vi "UpConvert.vi"(5 "clock x2":refnum<k21>="Daughterboard 0\\Data Clock x2", 7 "reset":bool, 8 "input valid":bool, 10 "output sample rate":fxp<+,48,1>, 11 "data in":T1[](array[typedef])=[{"I"=0.0, "Q"=0.0, "overflow"=FALSE}, {"I"=0.0, "Q"=0.0, "overflow"=FALSE}, {"I"=0.0, "Q"=0.0, "overflow"=FALSE}, {"I"=0.0, "Q"=0.0, "overflow"=FALSE}]) -> (0 "output valid":bool, 3 "data out":T1[](array[typedef]))   [LabVIEW 2025]
uses:
  <instrlib>/_niInstr/DSP/v1/FPGA/niInstr DSP v1 FPGA.lvlib
  <instrlib>/_niInstr/DSP/v1/Shared/Public/IQ Data.ctl
  <instrlib>/_niInstr/DSP/v1/Shared/niInstr DSP v1 Shared.lvlib
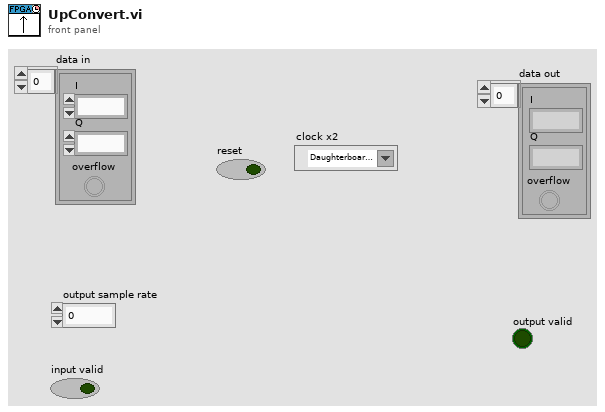
[diagram p1: front panel]
types:
  T1 = typedef "niInstr DSP v1 Shared.lvlib/IQ Data.ctl" = cluster{"I":fxp<+/-,18,1>, "Q":fxp<+/-,18,1>, "overflow":bool}
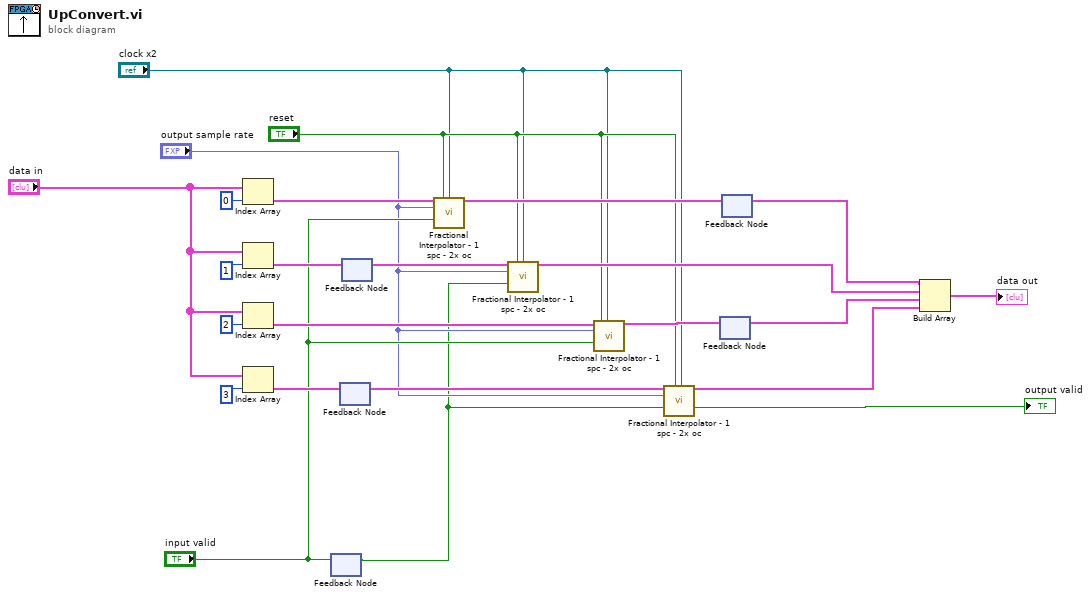
[diagram p0: block diagram]
diagram:
  n1 = Index Array(array="data in", index=0) -> (element=w14:T1)
  n2 = Index Array(array="data in", index=1) -> (element=w19:T1)
  n3 = Index Array(array="data in", index=2) -> (element=w10:T1)
  n4 = Index Array(array="data in", index=3) -> (element=w18:T1)
  n5 = feedback #1() -> (w5:bool)  [unwired: 1 in]
  n6 = feedback-in #1("input valid") -> ()
  n7 = feedback #2() -> (w7:T1)  [unwired: 1 in]
  n8 = feedback-in #2(w18) -> ()
  n9 = feedback #3() -> (w12:T1)  [unwired: 1 in]
  n10 = feedback-in #3(w19) -> ()
  n11 = call <instrlib>:"Fractional Interpolator - 1 spc - 2x oc.vi"("data in"=w14, "reset"="reset", "clock x 2"="clock x2", "input sample rate"="output sample rate", "input valid"="input valid") -> ("data out"=w13:T1)  [unwired: 7 in, 3 out]
  n12 = call <instrlib>:"Fractional Interpolator - 1 spc - 2x oc.vi"("data in"=w12, "reset"="reset", "clock x 2"="clock x2", "input sample rate"="output sample rate", "input valid"=w5) -> ("data out"=w11:T1)  [unwired: 7 in, 3 out]
  n13 = call <instrlib>:"Fractional Interpolator - 1 spc - 2x oc.vi"("data in"=w10, "reset"="reset", "clock x 2"="clock x2", "input sample rate"="output sample rate", "input valid"="input valid") -> ("data out"=w9:T1)  [unwired: 7 in, 3 out]
  n14 = call <instrlib>:"Fractional Interpolator - 1 spc - 2x oc.vi"("data in"=w7, "reset"="reset", "clock x 2"="clock x2", "input sample rate"="output sample rate", "input valid"=w5) -> ("data out"=w2:T1, "output valid"=→"output valid":bool)  [unwired: 7 in, 2 out]
  n15 = feedback #4() -> (w16:T1)  [unwired: 1 in]
  n16 = feedback-in #4(w9) -> ()
  n17 = feedback #5() -> (w17:T1)  [unwired: 1 in]
  n18 = feedback-in #5(w13) -> ()
  n19 = Build Array(w17, w11, w16, w2) -> (→"data out":T1[])
